vi "2-4040_Set SampleNumber&AcquireData1.vi"(8 "error in (no error)":errorcluster, 9 "WaveForm(3)":refnum<vi>[](array[refnum]), 10 "Sample Number":i32, 11 "VISA resource name":refnum<visa-resource-name>) -> (0 "error out":errorcluster, 1 "Pressure":dbl[](array[numeric]), 2 "Tem":dbl[](array[numeric]), 3 "Flow":dbl[](array[numeric]))   [LabVIEW 2017]
uses:
  <vilib>/Instr/_visa.llb/VISA Flush IO Buffer Mask.ctl
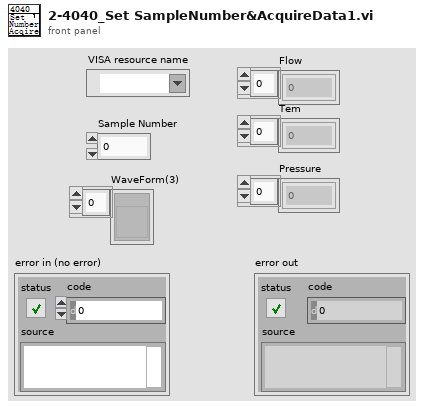
[diagram p1: front panel]
types:
  T1 = typedef "VISA Flush IO Buffer Mask.ctl" = u16
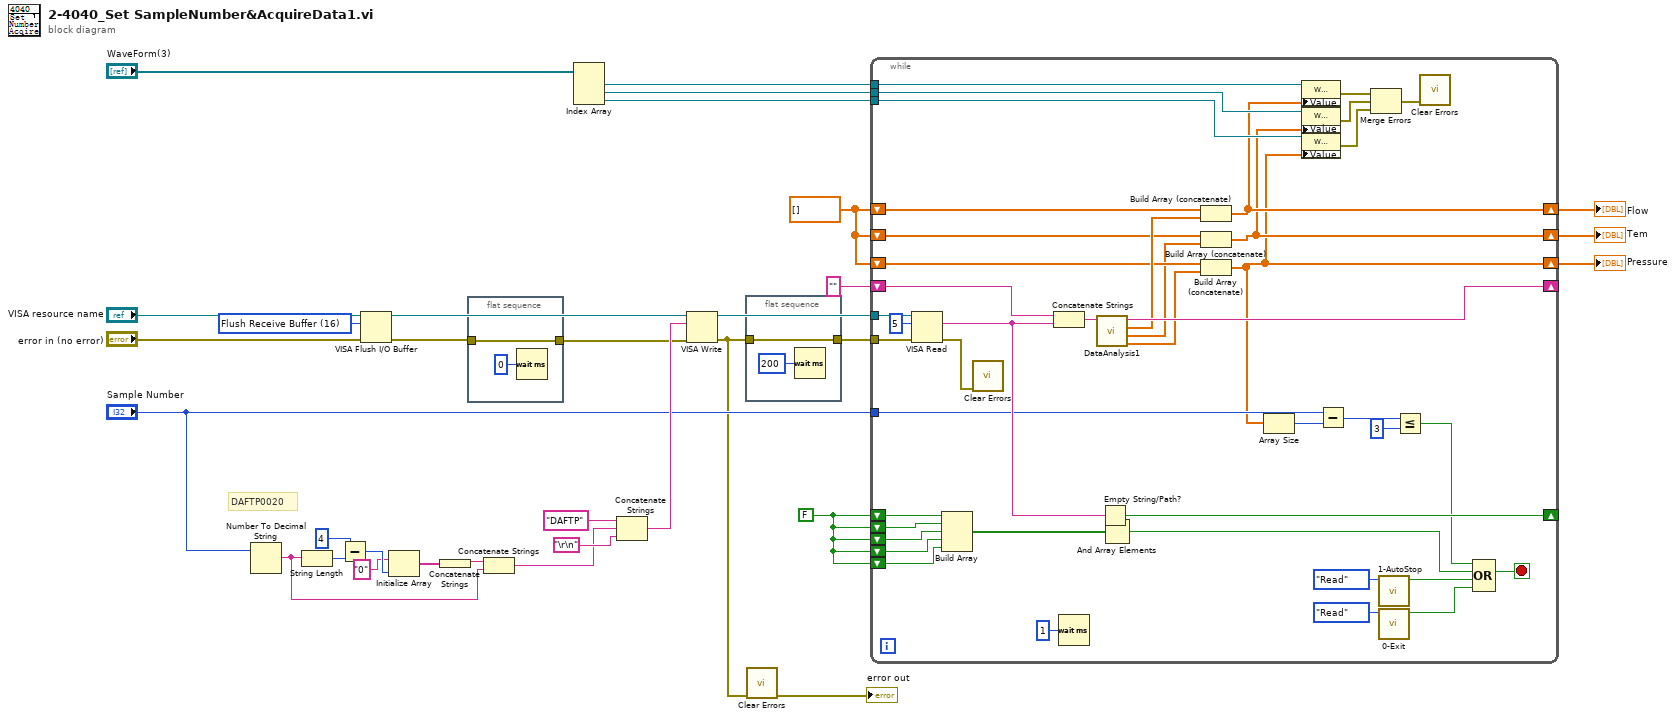
[diagram p0: block diagram]
diagram:
  w5 = T1 16 items=["Flush Receive Buffer"=16, "Write Transmit Buffer to Device"=32, "Flush Receive Buffer (No I/O)"=64, "Flush Transmit Buffer"=128] ("Mask")
  w12 = dbl[] []
  w15 = FALSE
  # "DAFTP0020"
  n1 = Number To Decimal String(number="Sample Number") -> (decimal integer string=w24:string)  [unwired: 1 in]
  n2 = String Length(string=w24) -> (length=w30:i32)
  n3 = Subtract(x=4, y=w30) -> (x-y=w28:i32)
  n4 = VISA Flush I/O Buffer(VISA resource name="VISA resource name", mask (16)=w5, error in (no error)="error in (no error)") -> (VISA resource name out=w7:refnum<visa-resource-name>, error out=w2:errorcluster)
  n5 = Initialize Array("0", w28) -> (w26:string[])
  n6 = Concatenate Strings(w26) -> (w25:string)
  n7 = flat-sequence {
    tunnel: w2 -> [w34]
    tunnel: [w34] -> w1
    frame #0 {
      n8 = Wait (ms)(milliseconds to wait=u32 0) -> ()  [unwired: 1 out]
    }
  }
  n9 = Concatenate Strings(w25, w24) -> (w23:string)
  n10 = Index Array(array="WaveForm(3)") -> (element #1=w18:refnum<vi>, element #2=w17:refnum<vi>, element #3=w16:refnum<vi>)  [unwired: 3 in]
  n11 = Concatenate Strings("DAFTP" ("写入缓冲区"), w23, "\r\n") -> (w22:string)
  n12 = VISA Write(VISA resource name=w7, write buffer=w22, error in (no error)=w1) -> (VISA resource name out=w21:refnum<visa-resource-name>, error out=w4:errorcluster)  [unwired: 1 out]
  n13 = flat-sequence {
    tunnel: w4 -> [w36]
    tunnel: [w36] -> w13
    frame #0 {
      n14 = Wait (ms)(milliseconds to wait=u32 200) -> ()  [unwired: 1 out]
    }
  }
  n15 = call <vilib>:"Clear Errors.vi"("error in (no error)"=w4) -> ("error out"=→"error out":errorcluster)  [unwired: 5 in, 1 out]
  n16 = while {
    tunnel: w13 -> [w78]
    tunnel: w21 -> [w79]
    shift-right: [w71] -> _
    shift-left: "" -> [w73]
    tunnel: w18 -> [w76]
    tunnel: w17 -> [w74]
    tunnel: w16 -> [w75]
    shift-right: [w68] -> _
    shift-left: w15 -> [w67]
    shift-left: w15 -> [w66]
    shift-left: w15 -> [w65]
    shift-left: w15 -> [w64]
    shift-left: w15 -> [w63]
    tunnel: "Sample Number" -> [w58]
    shift-right: [w39] -> w11
    shift-left: w12 -> [w55]
    shift-right: [w38] -> w10
    shift-left: w12 -> [w53]
    shift-right: [w37] -> w9
    shift-left: w12 -> [w52]
    stop <- w57 stop-if-true
    n17 = VISA Read(VISA resource name=w79, byte count=u32 5 ("字节总数"), error in (no error)=w78) -> (read buffer=w69:string, error out=w70:errorcluster)  [unwired: 2 out]
    n18 = Build Array(w67, w66, w65, w64, w63) -> (w62:bool[])
    n19 = call <vilib>:"Clear Errors.vi"("error in (no error)"=w70) -> ()  [unwired: 5 in, 2 out]
    n20 = Concatenate Strings(w73, w69) -> (w72:string)
    n21 = Wait (ms)(milliseconds to wait=u32 1) -> ()  [unwired: 1 out]
    n22 = call "DataAnalysis1.vi"("Data"=w72) -> ("3"=w50:dbl[], "2"=w51:dbl[], "1"=w54:dbl[], "Residue Datas"=w71:string)  [unwired: 7 in]
    n23 = Empty String/Path?(string/path=w69) -> (empty?=w68:bool)
    n24 = And Array Elements(Boolean array=w62) -> (logical AND=w61:bool)
    n25 = Build Array (concatenate)(w55, w54) -> (w39:dbl[])
    n26 = Build Array (concatenate)(w53, w51) -> (w38:dbl[])
    n27 = Build Array (concatenate)(w52, w50) -> (w37:dbl[])
    n28 = Array Size(array=w37) -> (size(s)=w45:i32)
    n29 = property class="WFGraph (strict)"(reference=w76, "Value"=w39) -> (error out=w49:errorcluster)  [unwired: 1 in, 1 out]
    n30 = property class="WFGraph (strict)"(reference=w74, "Value"=w38) -> (error out=w48:errorcluster)  [unwired: 1 in, 1 out]
    n31 = property class="WFGraph (strict)"(reference=w75, "Value"=w37) -> (error out=w47:errorcluster)  [unwired: 1 in, 1 out]
    n32 = Subtract(x=w58, y=w45) -> (x-y=w60:i32)
    n33 = Merge Errors(w49, w48, w47) -> (w46:errorcluster)
    n34 = call "1-AutoStop.vi"("Step"=enum16{"Initial", "Write", "Read"}."Read") -> ("AutoStop Out"=w41:bool)  [unwired: 9 in, 1 out]
    n35 = call "0-Exit.vi"("Step"=enum16{"Initial", "Write", "Read"}."Read") -> ("Exit Out"=w40:bool)  [unwired: 9 in, 1 out]
    n36 = Less Or Equal?(x=w60, y=3) -> (x <= y?=w56:bool)
    n37 = call <vilib>:"Clear Errors.vi"("error in (no error)"=w46) -> ()  [unwired: 5 in, 2 out]
    n38 = Compound Arithmetic op=OR(w56, w61, w41, w40) -> (w57:bool)
  }
  "Flow" <- w11
  "Tem" <- w10
  "Pressure" <- w9
